vi "mlog3.vi"(1 "error in":errorcluster) -> (0 "message":string)   [LabVIEW 2010]
uses:
  <vilib>/Utility/error.llb/DialogType.ctl
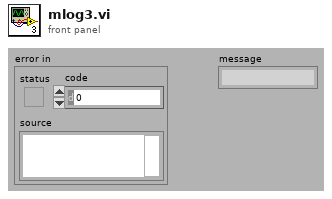
[diagram p1: front panel]
types:
  T1 = typedef "DialogType.ctl" = u16
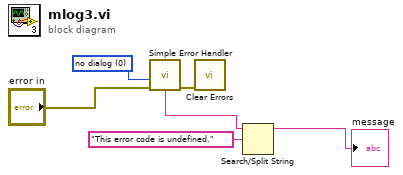
[diagram p0: block diagram]
diagram:
  w3 = T1 0 items=["no dialog", "OK message", "continue or stop message", "OK message + warnings", "continue/stop + warnings"] ("type of dialog (OK msg:1)")
  n1 = call <vilib>:"Simple Error Handler.vi"("type of dialog (OK msg:1)"=w3, "error in (no error)"="error in") -> ("error out"=w2:errorcluster, "message"=w5:string)  [unwired: 3 in, 3 out]
  n2 = call <vilib>:"Clear Errors.vi"("error in (no error)"=w2) -> ()  [unwired: 6 in, 1 out]
  n3 = Search/Split String(string=w5, search string/char (-)="This error code is undefined.") -> (substring before match=→"message":string)  [unwired: 1 in, 2 out]
